vi "PRO_Check ValuesV1.vi"(6 "error in (no error)":errorcluster, 8 "Results in":T3=[[{"Fill"=0.0, "Drain"=7.150000000000002, "Status"=9, "Resistor"=100.0}, {"Fill"=0.0, "Drain"=6.925000000000003, "Status"=9, "Resistor"=100.0}], [{"Fill"=7.1350000000000025, "Drain"=6.700000000000004, "Status"=9, "Resistor"=200.0}, {"Fill"=6.910000000000004, "Drain"=6.475000000000005, "Status"=9, "Resistor"=200.0}], [{"Fill"=6.685000000000004, "Drain"=6.250000000000005, "Status"=9, "Resistor"=300.0}, {"Fill"=6.460000000000004, "Drain"=6.025000000000006, "Status"=9, "Resistor"=300.0}], [{"Fill"=6.235000000000006, "Drain"=5.8000000000000025, "Status"=9, "Resistor"=400.0}, {"Fill"=6.010000000000005, "Drain"=5.59, "Status"=9, "Resistor"=400.0}], [{"Fill"=5.785000000000002, "Drain"=5.364999999999997, "Status"=9, "Resistor"=500.0}, {"Fill"=5.574999999999999, "Drain"=5.1399999999999935, "Status"=9, "Resistor"=500.0}], [{"Fill"=5.349999999999996, "Drain"=4.91499999999999, "Status"=9, "Resistor"=600.0}, {"Fill"=5.124999999999993, "Drain"=4.689999999999987, "Status"=9, "Resistor"=600.0}], [{"Fill"=4.89999999999999, "Drain"=4.464999999999983, "Status"=9, "Resistor"=700.0}, {"Fill"=4.6749999999999865, "Drain"=4.23999999999998, "Status"=9, "Resistor"=700.0}], [{"Fill"=4.449999999999983, "Drain"=4.014999999999977, "Status"=9, "Resistor"=800.0}, {"Fill"=4.22499999999998, "Drain"=3.7899999999999734, "Status"=9, "Resistor"=800.0}], [{"Fill"=3.999999999999977, "Drain"=3.56499999999997, "Status"=9, "Resistor"=900.0}, {"Fill"=3.7749999999999737, "Drain"=3.339999999999967, "Status"=9, "Resistor"=900.0}], [{"Fill"=3.5499999999999705, "Drain"=3.114999999999964, "Status"=9, "Resistor"=1000.0}, {"Fill"=3.3249999999999673, "Drain"=2.8899999999999606, "Status"=9, "Resistor"=1000.0}], [{"Fill"=3.099999999999964, "Drain"=0.0, "Status"=5, "Resistor"=1100.0}, {"Fill"=2.874999999999961, "Drain"=0.0, "Status"=5, "Resistor"=1100.0}]] {"Resistor" format="%.1f"; "Drain" format="%.3f"; "Fill" format="%.3f"}, 10 "aSpec In":T1[](array[typedef]), 11 "Measurement":T4=[{"Switched"=FALSE, "In Range"=TRUE, "Index"=1, "Level OUt"=8.485, " Ch n Ohms"=100.0, "Drain!Fill"=FALSE}, {"Switched"=FALSE, "In Range"=TRUE, "Index"=1, "Level OUt"=8.485, " Ch n Ohms"=100.0, "Drain!Fill"=FALSE}]) -> (0 "Results out":T3=[[{"Fill"=0.0, "Drain"=7.150000000000002, "Status"=9, "Resistor"=100.0}, {"Fill"=0.0, "Drain"=6.925000000000003, "Status"=9, "Resistor"=100.0}], [{"Fill"=7.1350000000000025, "Drain"=6.700000000000004, "Status"=9, "Resistor"=200.0}, {"Fill"=6.910000000000004, "Drain"=6.475000000000005, "Status"=9, "Resistor"=200.0}], [{"Fill"=6.685000000000004, "Drain"=6.250000000000005, "Status"=9, "Resistor"=300.0}, {"Fill"=6.460000000000004, "Drain"=6.025000000000006, "Status"=9, "Resistor"=300.0}], [{"Fill"=6.235000000000006, "Drain"=5.8000000000000025, "Status"=9, "Resistor"=400.0}, {"Fill"=6.010000000000005, "Drain"=5.59, "Status"=9, "Resistor"=400.0}], [{"Fill"=5.785000000000002, "Drain"=5.364999999999997, "Status"=9, "Resistor"=500.0}, {"Fill"=5.574999999999999, "Drain"=5.1399999999999935, "Status"=9, "Resistor"=500.0}], [{"Fill"=5.349999999999996, "Drain"=4.91499999999999, "Status"=9, "Resistor"=600.0}, {"Fill"=5.124999999999993, "Drain"=4.689999999999987, "Status"=9, "Resistor"=600.0}], [{"Fill"=4.89999999999999, "Drain"=4.464999999999983, "Status"=9, "Resistor"=700.0}, {"Fill"=4.6749999999999865, "Drain"=4.23999999999998, "Status"=9, "Resistor"=700.0}], [{"Fill"=4.449999999999983, "Drain"=4.014999999999977, "Status"=9, "Resistor"=800.0}, {"Fill"=4.22499999999998, "Drain"=3.7899999999999734, "Status"=9, "Resistor"=800.0}], [{"Fill"=3.999999999999977, "Drain"=3.56499999999997, "Status"=9, "Resistor"=900.0}, {"Fill"=3.7749999999999737, "Drain"=3.339999999999967, "Status"=9, "Resistor"=900.0}], [{"Fill"=3.5499999999999705, "Drain"=3.114999999999964, "Status"=9, "Resistor"=1000.0}, {"Fill"=3.3249999999999673, "Drain"=2.8899999999999606, "Status"=9, "Resistor"=1000.0}], [{"Fill"=3.099999999999964, "Drain"=0.0, "Status"=5, "Resistor"=1100.0}, {"Fill"=2.874999999999961, "Drain"=0.0, "Status"=5, "Resistor"=1100.0}]] {"Resistor" format="%.1f"; "Drain" format="%.3f"; "Fill" format="%.3f"}, 1 "Err Num":i32, 4 "error out":errorcluster)   [LabVIEW 2024]
uses:
  Control Definitions/Def Xresult.ctl
  Control Definitions/Def Results2.ctl
  Control Definitions/Ded Spec RNG.ctl
  Control Definitions/Ded LUT_Status.ctl
panel:
  # "ChA=0; ChB=1"
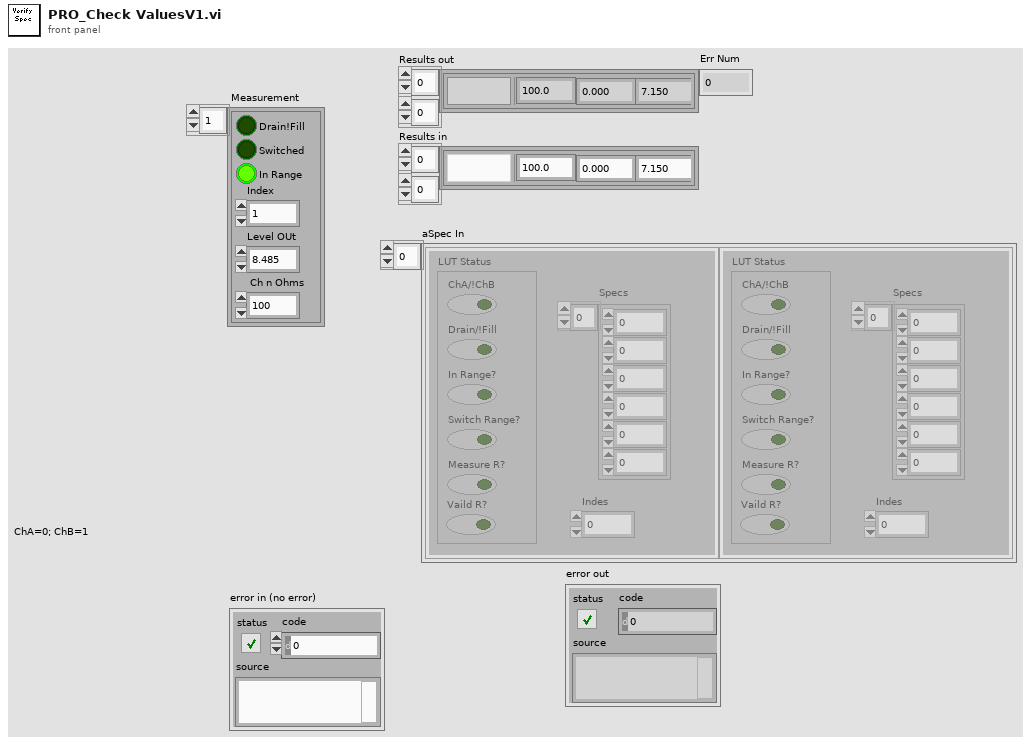
[diagram p1: front panel]
types:
  T1 = typedef "Ded Spec RNG.ctl" = cluster{"Specs":dbl[], "Indes":i32, "LUT Status":T2}
  T2 = typedef "Ded LUT_Status.ctl" = cluster{"ChA/!ChB":bool, "Drain/!Fill":bool, "In Range?":bool, "Switch Range?":bool, "Measure R?":bool, "Vaild R?":bool}
  T3 = typedef "Def Results2.ctl" = cluster{"Fill":dbl, "Drain":dbl, "Status":i16, "Resistor":dbl}[][]
  T4 = typedef "Def Xresult.ctl" = cluster{"Switched":bool, "In Range":bool, "Index":i16, "Level OUt":dbl, " Ch n Ohms":dbl, "Drain!Fill":bool}[]
  T5 = cluster{"Fill":dbl, "Drain":dbl, "Status":i16, "Resistor":dbl}
  T6 = cluster{"Switched":bool, "In Range":bool, "Index":i16, "Level OUt":dbl, " Ch n Ohms":dbl, "Drain!Fill":bool}
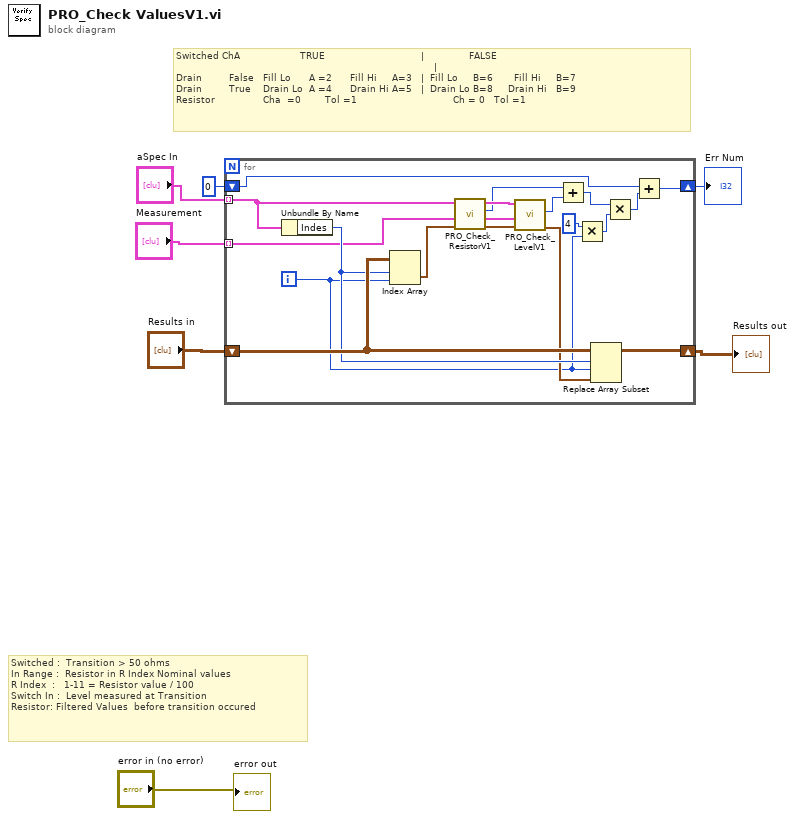
[diagram p0: block diagram]
diagram:
  # "Switched ChA                    TRUE                                |               FALSE\n                                                                                      |\nDrain         False   Fill Lo      A =2      Fill Hi     A=3   |  Fill Lo     B=6       Fill Hi     B=7\nDrain         True    Drain Lo  A =4      Drain Hi A=5   |  Drain Lo B=8     Drain Hi   B=9 \nResistor                Cha  =0        Tol =1                                Ch = 0   Tol =1"
  # "Switched :  Transition > 50 ohms\nIn Range :  Resistor in R Index Nominal values\nR Index  :   1-11 = Resistor value / 100\nSwitch In :  Level measured at Transition\nResistor: Filtered Values  before transition occured"
  n1 = for {
    tunnel: "aSpec In" -> [w23] mode=indexing
    tunnel: "Measurement" -> [w22] mode=indexing
    shift-right: [w24] -> w3
    shift-left: "Results in" -> [w26]
    shift-right: [w10] -> w1
    shift-left: 0 -> [w9]
    i -> [w14]
    n2 = Unbundle By Name(w23) -> ("Indes"=w25:i32)
    n3 = Index Array(array=w26, index (row)=w25, index (col)=w14) -> (element=w21:T5)
    n4 = call "PRO_Check_ResistorV1.vi"("Results In"=w21, "Measure in"=w22, "ChA Spec RNG In"=w23) -> ("Results out"=w18:T5, "Measure Out"=w19:T6, "Err Num"=w15:i32, "ChA Spec RNG Out"=w20:T1)  [unwired: 4 in]
    n5 = call "PRO_Check_LevelV1.vi"("Results in"=w18, "Measure In"=w19, "ChA Spec RNG In"=w20) -> ("Results out"=w17:T5, "Err Num"=w16:i32)  [unwired: 7 in]
    n6 = Add(x=w15, y=w16) -> (x+y=w12:i32)
    n7 = Multiply(x=4, y=w14) -> (x*y=w13:i32)
    n8 = Replace Array Subset(array=w26, new element=w17, index (row)=w25, index (col)=w14) -> (w24:T3)
    n9 = Multiply(x=w12, y=w13) -> (x*y=w11:i32)
    n10 = Add(x=w9, y=w11) -> (x+y=w10:i32)
  }
  "Results out" <- w3
  "Err Num" <- w1
  "error out" <- "error in (no error)"
